vi "ce14. cos phi.vi"(8 "error in (no error)":errorcluster, 10 "kvar":dbl, 11 "kW":dbl=1.0) -> (0 "error out":errorcluster, 3 "cos phi":dbl)   [LabVIEW 2018, in "CE14_eMIC.lvlib"]
uses:
  CE14_eMIC.lvlib
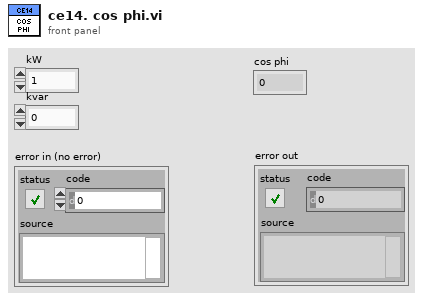
[diagram p1: front panel]
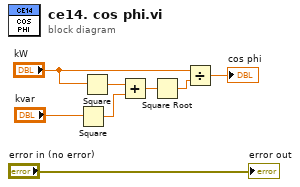
[diagram p0: block diagram]
diagram:
  n1 = Square(x="kvar") -> (x^2=w6:dbl)
  n2 = Square(x="kW") -> (x^2=w7:dbl)
  n3 = Add(x=w7, y=w6) -> (x+y=w5:dbl)
  n4 = Square Root(x=w5) -> (sqrt(x)=w4:dbl)
  n5 = Divide(x="kW", y=w4) -> (x/y=→"cos phi":dbl)
  "error out" <- "error in (no error)"
